vi "文件格式化写入.vi"() -> ()   [LabVIEW 2018]
panel:
  out "错误输出":errorcluster
  in  "停止":bool
  in  "确定按钮":bool
  out "错误输出 2":errorcluster caption="错误输出"
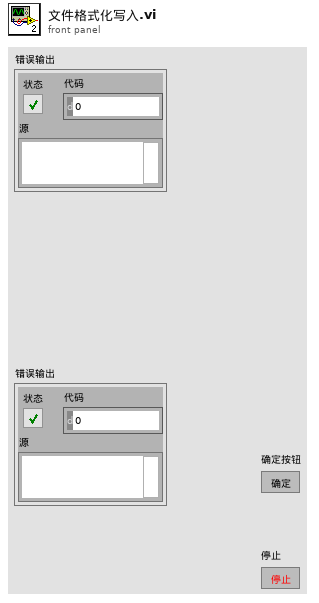
[diagram p1: front panel]
types:
  T1 = enum16{"open", "replace", "create", "open or create", "replace or create", "replace or create with confirmation"}
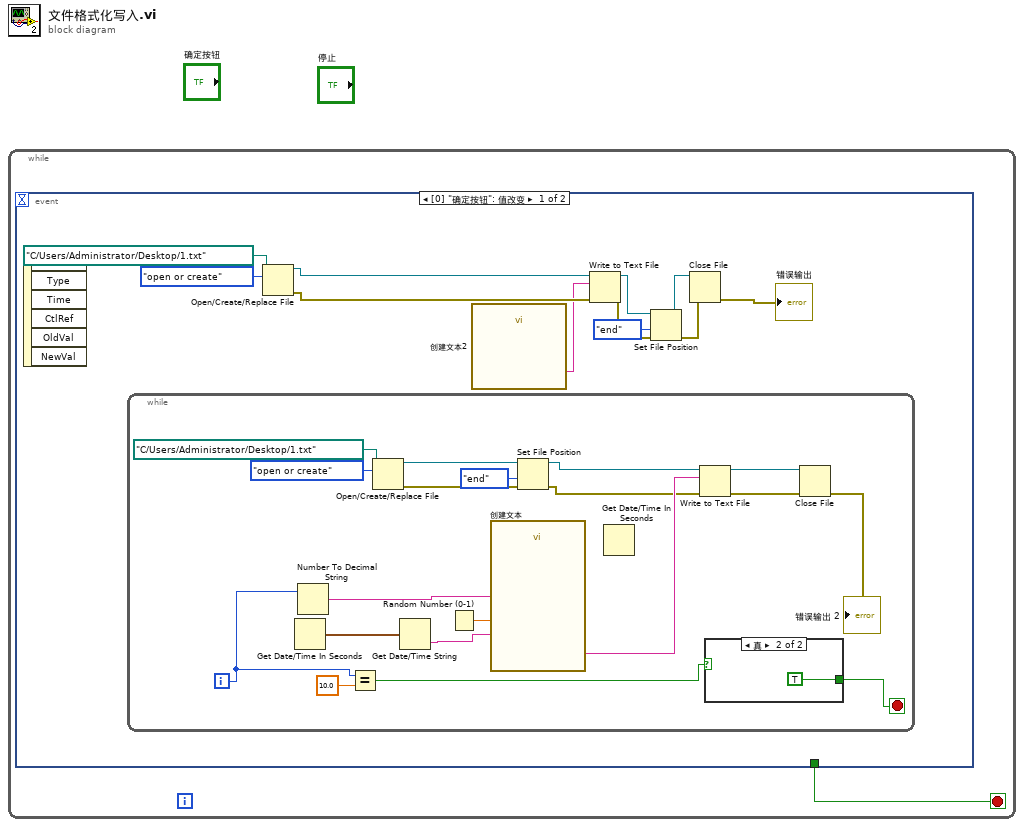
[diagram p0: block diagram]
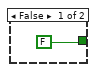
[diagram p2: hidden frame]
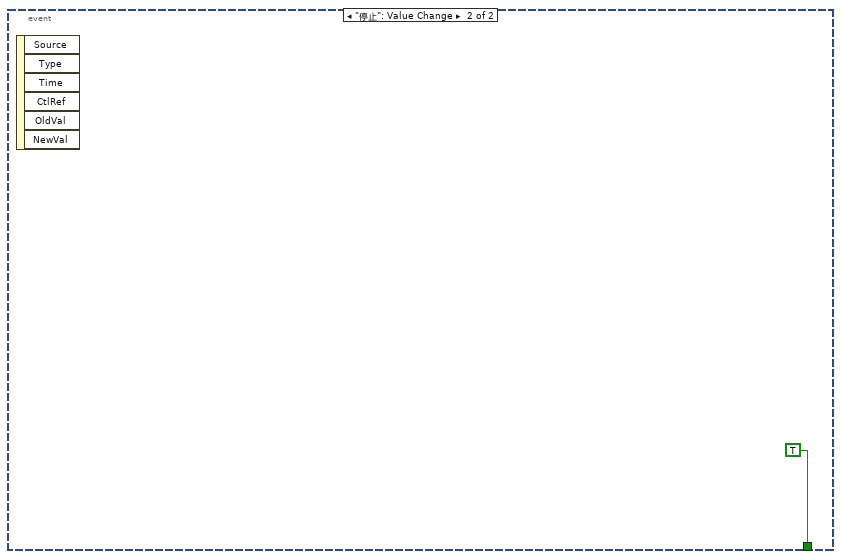
[diagram p3: hidden frame]
diagram:
  n1 = while {
    stop <- w1 stop-if-true
    n2 = event shown="[0] \"确定按钮\": 值改变" {
      selector: _ -> [_ _]
      dyn-events: _ -> [_ _]
      timeout: _ -> [_ _]
      tunnel: [_ TRUE] -> w1
      event "确定按钮": Value Change {
        n3 = event-data() -> ()  [unwired: 1 in, 6 out]
        n4 = while {
          i -> [w26]
          stop <- w24 stop-if-true
          n5 = Get Date/Time In Seconds() -> (seconds since 1Jan1904=w30:timestamp)
          n6 = Number To Decimal String(number=w26) -> (decimal integer string=w23:string)  [unwired: 1 in]
          n7 = Equal?(x=w26, y=10.0) -> (x = y?=w25:bool)
          n8 = Open/Create/Replace File(file path (use dialog)=path "C:/Users/Administrator/Desktop/1.txt" ("文件路径（使用对话框）"), operation (0:open)=T1."open or create" ("操作(0:open)")) -> (refnum out=w17:refnum<file>, error out=w15:errorcluster)  [unwired: 4 in, 1 out]
          n9 = Get Date/Time String(seconds (now)=w30) -> (time string=w22:string)  [unwired: 2 in, 1 out]
          n10 = Random Number (0-1)() -> (number: 0 to 1=w18:dbl)
          n11 = call "创建文本"("a"=w23, "b"=w18, "c"=w22) -> ("Result"=w21:string)  [unwired: 11 in, 1 out]
          n12 = Set File Position(refnum=w17, from (0:start)=enum16{"start", "end", "current"}."end" ("自（0:起始）"), error in=w15) -> (refnum out=w16:refnum<file>, error out=w14:errorcluster)  [unwired: 1 in]
          n13 = Get Date/Time In Seconds() -> ()  [unwired: 1 out]
          n14 = Write to Text File(file (use dialog)=w16, text=w21, error in=w14) -> (refnum out=w20:refnum<file>, error out=w19:errorcluster)  [unwired: 1 in, 1 out]
          n15 = case shown="真" w25 {
            tunnel: [FALSE TRUE] -> w24
            frame False {
            }
            frame True {
            }
          }
          n16 = Close File(refnum=w20, error in=w19) -> (error out=→"错误输出 2":errorcluster)  [unwired: 1 out]
        }
        n17 = Open/Create/Replace File(file path (use dialog)=path "C:/Users/Administrator/Desktop/1.txt" ("文件路径（使用对话框）"), operation (0:open)=T1."open or create" ("操作(0:open)")) -> (refnum out=w10:refnum<file>, error out=w9:errorcluster)  [unwired: 4 in, 1 out]
        n18 = call "创建文本2"() -> ("Result"=w8:string)  [unwired: 14 in, 1 out]
        n19 = Write to Text File(file (use dialog)=w10, text=w8, error in=w9) -> (refnum out=w6:refnum<file>, error out=w4:errorcluster)  [unwired: 1 in, 1 out]
        n20 = Set File Position(refnum=w6, from (0:start)=enum16{"start", "end", "current"}."end" ("自（0:起始）"), error in=w4) -> (refnum out=w5:refnum<file>, error out=w3:errorcluster)  [unwired: 1 in]
        n21 = Close File(refnum=w5, error in=w3) -> (error out=→"错误输出":errorcluster)  [unwired: 1 out]
      }
      event "停止": Value Change {
        n22 = event-data() -> ()  [unwired: 1 in, 6 out]
      }
    }
  }
